vi "_Counter-Increment.vi"(6 "LIBNAME":string, 7 "VI Refnum":refnum<vi>, 8 "error in (no error)":errorcluster, 10 "name(\"\")":string) -> (0 "error out":errorcluster, 2 "cacher":T1, 3 "queue out":T2)   [LabVIEW 2017, in "StopSignal.lvlib"]
uses:
  StopSignal.lvlib
  Typedef/StopSignal.ctl
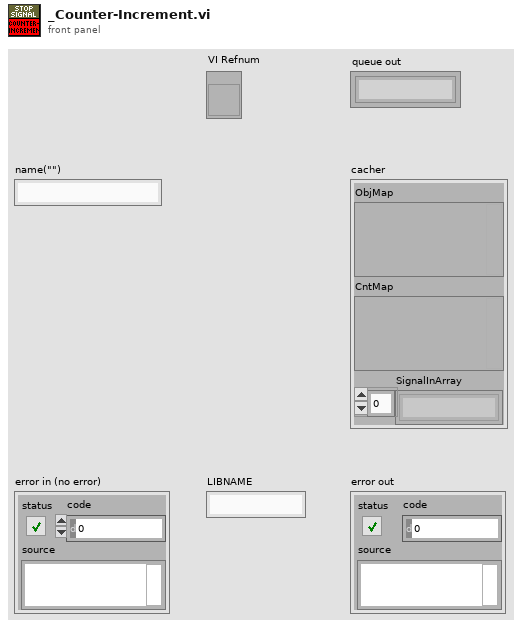
[diagram p1: front panel]
types:
  T1 = cluster{"ObjMap":variant, "CntMap":variant, "SignalInArray":string[]}
  T2 = typedef "StopSignal.lvlib/StopSignal.ctl" = refnum<k1>
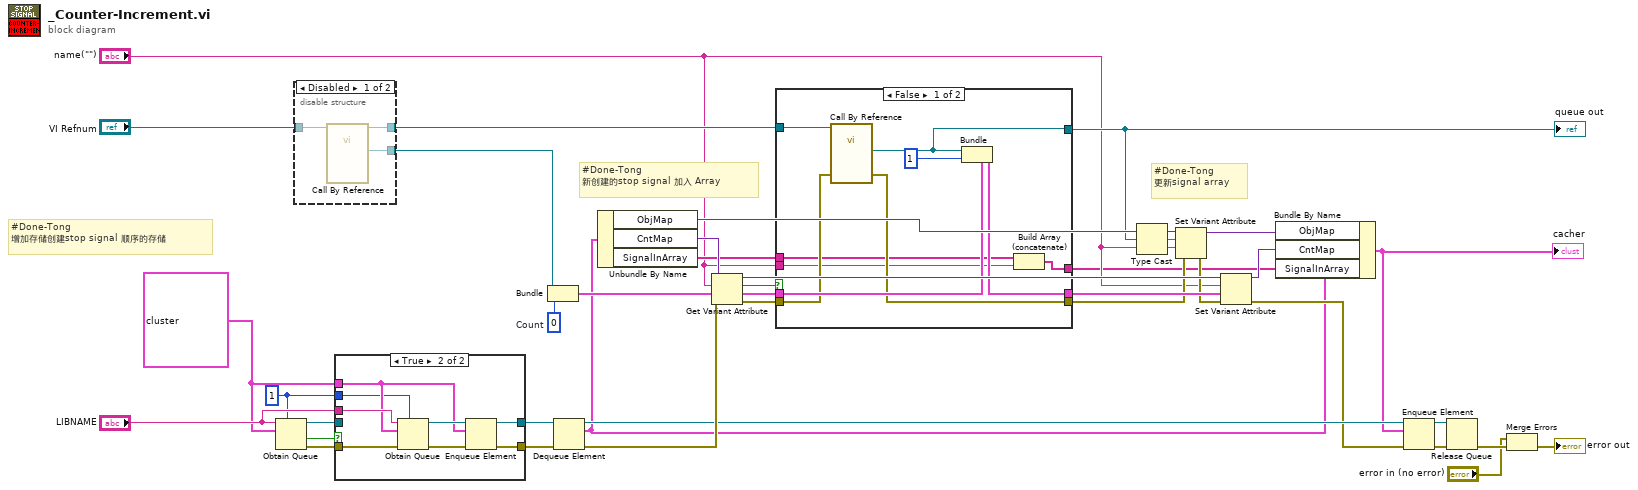
[diagram p0: block diagram]
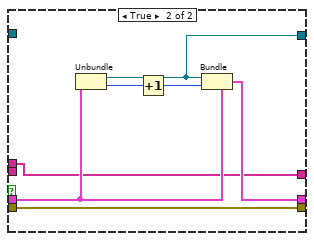
[diagram p3: hidden frame]
diagram:
  w14 = 1 ("max queue size (-1, unlimited)")
  w15 = T1 {"ObjMap"=variant, "CntMap"=variant, "SignalInArray"=[]}
  w23 = 0  # Count
  # "#Done-Tong\n更新signal array"
  # "#Done-Tong\n新创建的stop signal 加入 Array"
  # "#Done-Tong\n增加存储创建stop signal 顺序的存储"
  n1 = Obtain Queue(max queue size (-1, unlimited)=w14, name (unnamed)="LIBNAME", element data type=w15) -> (queue out=w36:refnum<queue>, created new?=w38:bool, error out=w37:errorcluster)  [unwired: 2 in]
  n2 = disable-structure shown="Disabled" {
    disable-tunnel: "VI Refnum" -> [w42 w43]
    disable-tunnel: [w41 _] -> w21
    disable-tunnel: [w40 w43] -> w20
    frame Disabled {
      n3 = call-by-ref "?"(reference=w42) -> (reference out=w40:refnum<vi>, "StopSignal"=w41:T2)  [unwired: 11 in, 2 out]
    }
    frame Enabled {
    }
  }
  n4 = case shown="True" w38 {
    tunnel: w37 -> [w44 w51]
    tunnel: w36 -> [w45 _]
    tunnel: w15 -> [_ w47]
    tunnel: [w44 w53] -> w35
    tunnel: [w45 w52] -> w34
    tunnel: "LIBNAME" -> [_ w48]
    tunnel: w14 -> [_ w46]
    frame False {
    }
    frame True {
      n5 = Obtain Queue(max queue size (-1, unlimited)=w46, name (unnamed)=w48, element data type=w47, error in (no error)=w51) -> (queue out=w49:refnum<queue>, error out=w50:errorcluster)  [unwired: 1 in, 1 out]
      n6 = Enqueue Element(queue=w49, element=w47, error in (no error)=w50) -> (queue out=w52:refnum<queue>, error out=w53:errorcluster)  [unwired: 1 in, 1 out]
    }
  }
  n7 = Bundle("StopSignal"=w21, "Count"=w23) -> (w22:cluster{"StopSignal":T2, "Count":i32})  [unwired: 1 in]
  n8 = Dequeue Element(queue=w34, error in (no error)=w35) -> (queue out=w28:refnum<queue>, element=w12:T1, error out=w33:errorcluster)  [unwired: 1 in, 1 out]
  n9 = Unbundle By Name(w12) -> ("ObjMap"=w7:variant, "CntMap"=w13:variant, "SignalInArray"=w4:string[])
  n10 = Get Variant Attribute(Variant=w13, name="name(\"\")", default value (empty Variant)=w22, error in=w33) -> (duplicate Variant=w30:variant, found=w32:bool, value=w31:cluster{"StopSignal":T2, "Count":i32}, error out=w25:errorcluster)
  n11 = case shown="False" w32 {
    tunnel: w31 -> [w63 w70]
    tunnel: [w61 w69] -> w29
    tunnel: [w57 w68] -> w6
    tunnel: w25 -> [w59 w67]
    tunnel: [w58 w67] -> w9
    tunnel: w20 -> [w60 _]
    tunnel: w4 -> [w56 w64]
    tunnel: "name(\"\")" -> [w55 _]
    tunnel: [w54 w64] -> w2
    frame False {
      n12 = call-by-ref "?"(reference=w60, "error in (no error)"=w59) -> ("error out"=w58:errorcluster, "StopSignal"=w57:T2)  [unwired: 10 in, 2 out]
      n13 = Bundle(cluster=w63, "StopSignal"=w57, "Count"=1) -> (w61:cluster{"StopSignal":T2, "Count":i32})
      n14 = Build Array (concatenate)(w56, w55) -> (w54:string[])
    }
    frame True {
      n15 = Unbundle(w70) -> ("StopSignal"=w68:T2, "Count"=w66:i32)
      n16 = Increment(x=w66) -> (x+1=w65:i32)
      n17 = Bundle(cluster=w70, "StopSignal"=w68, "Count"=w65) -> (w69:cluster{"StopSignal":T2, "Count":i32})
    }
  }
  "queue out" <- w6
  n18 = Type Cast(x=w6) -> (*(type *) &x=w5:string)  [unwired: 1 in]
  n19 = Set Variant Attribute(Variant=w7, name=w5, value="name(\"\")", error in=w9) -> (Variant out=w10:variant, error out=w8:errorcluster)  [unwired: 1 out]
  n20 = Set Variant Attribute(Variant=w30, name="name(\"\")", value=w29, error in=w8) -> (Variant out=w11:variant, error out=w24:errorcluster)  [unwired: 1 out]
  n21 = Bundle By Name(cluster=w12, "ObjMap"=w10, "CntMap"=w11, "SignalInArray"=w2) -> (w1:T1)
  "cacher" <- w1
  n22 = Enqueue Element(queue=w28, element=w1, error in (no error)=w24) -> (queue out=w27:refnum<queue>, error out=w26:errorcluster)  [unwired: 1 in, 1 out]
  n23 = Release Queue(queue=w27, error in (no error)=w26) -> (error out=w39:errorcluster)  [unwired: 1 in, 2 out]
  n24 = Merge Errors("error in (no error)", w39) -> (→"error out":errorcluster)
